vi "Build Control Word.vi"(7 "Virtual Memory Unit in":refnum<class "Virtual Memory Unit.lvclass">, 8 "error in (no error)":errorcluster, 10 "Starting Address":u16 format="%04x", 11 "Message in":refnum<class "Message.lvclass">) -> (0 "error out":errorcluster, 2 "Next Available Address":u16 format="%04x", 3 "Message out":refnum<class "Message.lvclass">, 5 "Virtual Memory Unit out":refnum<class "Virtual Memory Unit.lvclass">)   [LabVIEW 2020, in "BCI-1553 API.lvlib" / "Message.lvclass"]
doc: "Builds the BC Control word for this message and places it into virtual memory."
uses:
  Message.lvclass
  Dependencies/Virtual Memory Unit/Virtual Memory Unit.lvclass
  Message.lvclass/Message.ctl
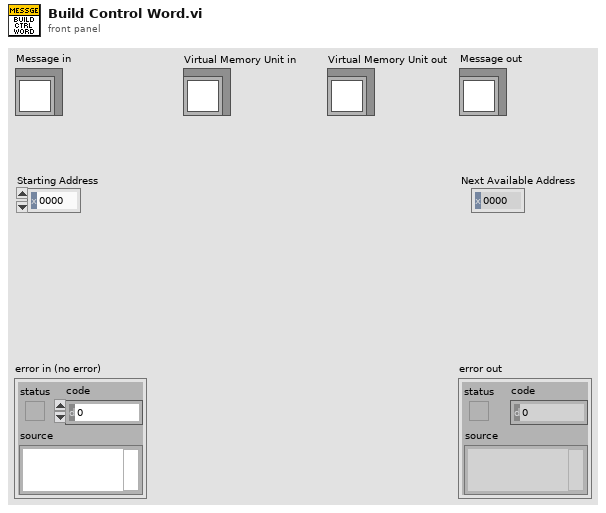
[diagram p1: front panel]
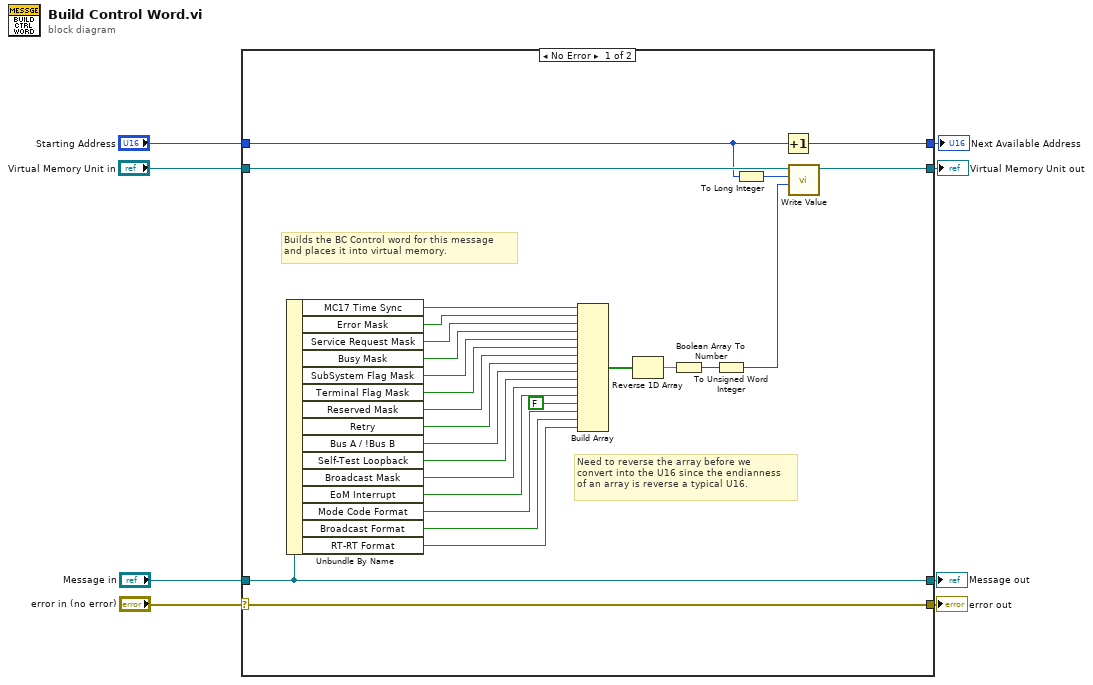
[diagram p0: block diagram]
diagram:
  n1 = case shown="No Error" "error in (no error)" {
    selector: "error in (no error)" -> [w35 w39]
    tunnel: [w35 w39] -> w7
    tunnel: [w34 w38] -> w5
    tunnel: "Message in" -> [w34 w38]
    tunnel: "Virtual Memory Unit in" -> [w13 w36]
    tunnel: "Starting Address" -> [w10 w37]
    tunnel: [w33 w37] -> w2
    tunnel: [w12 w36] -> w1
    frame No Error {
      # "Need to reverse the array before we\nconvert into the U16 since the endianness\nof an array is reverse a typical U16."
      # "Builds the BC Control word for this message\nand places it into virtual memory."
      n2 = Unbundle By Name(w34) -> ("MC17 Time Sync"=w14:bool, "Error Mask"=w20:bool, "Service Request Mask"=w21:bool, "Busy Mask"=w22:bool, "SubSystem Flag Mask"=w23:bool, "Terminal Flag Mask"=w24:bool, "Reserved Mask"=w25:bool, "Retry"=w26:bool, "Bus A / !Bus B"=w27:bool, "Self-Test Loopback"=w28:bool, "Broadcast Mask"=w29:bool, "EoM Interrupt"=w18:bool, "Mode Code Format"=w19:bool, "Broadcast Format"=w32:bool, "RT-RT Format"=w31:bool)
      n3 = Build Array(w14, w20, w21, w22, w23, w24, w25, w26, w27, w28, w29, w18, FALSE ("element"), w19, w32, w31) -> (w17:bool[])
      n4 = Reverse 1D Array(array=w17) -> (reversed array=w16:bool[])
      n5 = Boolean Array To Number(Boolean array=w16) -> (number=w15:u32)
      n6 = To Unsigned Word Integer(number=w15) -> (unsigned 16bit integer=w9:u16)
      n7 = To Long Integer(number=w10) -> (32bit integer=w11:i32)
      n8 = Increment(x=w10) -> (x+1=w33:u16)
      n9 = call "Write Value.vi"("Value"=w9, "Index"=w11, "Virtual Memory Unit in"=w13) -> ("Virtual Memory Unit out"=w12:refnum<class "Virtual Memory Unit.lvclass">)  [unwired: 7 in, 1 out]
    }
    frame Error {
    }
  }
  "error out" <- w7
  "Message out" <- w5
  "Virtual Memory Unit out" <- w1
  "Next Available Address" <- w2
